vi "FPGA EX.vi"() -> ()   [LabVIEW 2014]
uses:
  <vilib>/rvi/Emulation/niFpgaGetClockAttributes.vi
  <vilib>/rvi/Emulation/niFpgaSctlEmulationGetInTimedLoop.vi
  <vilib>/rvi/Emulation/niFpgaEmulationReportErrorSimple.vi
  <vilib>/rvi/eio/common/nirviEmuTemplateMethod_errors.vi
  <vilib>/rvi/Emulation/niFpgaCriticalErrorInLSC.vi
  <vilib>/eio/EIONode/EIONode.xnode
panel:
  in  "Mod4/AO2":fxp<+/-,20,5>
  in  "Mod4/AO3":fxp<+/-,20,5>
  in  "Mod4/AO1":fxp<+/-,20,5>
  in  "Mod4/AO0":fxp<+/-,20,5>
  out "Mod3/AI5":fxp<+/-,16,5>
  out "Mod3/AI3":fxp<+/-,16,5>
  out "Mod3/AI7":fxp<+/-,16,5>
  out "Mod3/AI6":fxp<+/-,16,5>
  out "Mod3/AI4":fxp<+/-,16,5>
  out "Mod3/AI2":fxp<+/-,16,5>
  out "Mod3/AI1":fxp<+/-,16,5>
  out "Mod3/AI0":fxp<+/-,16,5>
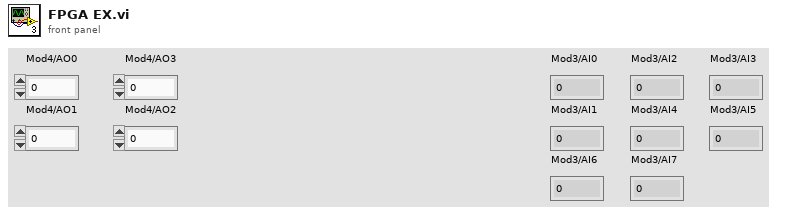
[diagram p1: front panel]
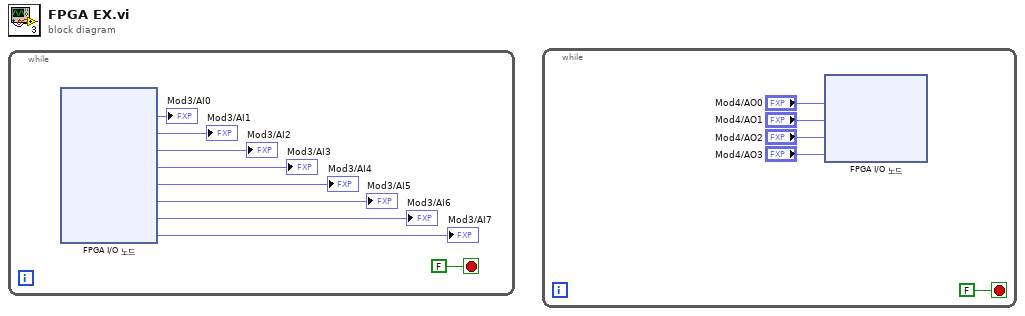
[diagram p0: block diagram]
diagram:
  n1 = while {
    stop <- FALSE stop-if-true
    n2 = xnode "FPGA I/O 노드"() -> ("Mod3/AI0"=→"Mod3/AI0":fxp<+/-,16,5>, "Mod3/AI1"=→"Mod3/AI1":fxp<+/-,16,5>, "Mod3/AI2"=→"Mod3/AI2":fxp<+/-,16,5>, "Mod3/AI3"=→"Mod3/AI3":fxp<+/-,16,5>, "Mod3/AI4"=→"Mod3/AI4":fxp<+/-,16,5>, "Mod3/AI5"=→"Mod3/AI5":fxp<+/-,16,5>, "Mod3/AI6"=→"Mod3/AI6":fxp<+/-,16,5>, "Mod3/AI7"=→"Mod3/AI7":fxp<+/-,16,5>)  [unwired: 8 in, 8 out]
  }
  n3 = while {
    stop <- FALSE stop-if-true
    n4 = xnode "FPGA I/O 노드"("Mod4/AO0"="Mod4/AO0", "Mod4/AO1"="Mod4/AO1", "Mod4/AO2"="Mod4/AO2", "Mod4/AO3"="Mod4/AO3") -> ()  [unwired: 4 in, 4 out]
  }
